vi "Reset Front Panel.vi"(7 "Active Display":u16, 8 "error in":errorcluster, 9 "Pane Origin":T1[](array[typedef]), 10 "Front Panel Bounds":T2, 11 "VI Ref":refnum<vi>) -> (0 "error out":errorcluster, 3 "VI Ref":refnum<vi>)   [LabVIEW 2014]
doc: "<B>Copyright</B>: (c) 2015 MHWirth. All rights reserved.\n\nThis subVI retreive the front panel size and organization. \nThis can be called in \"Panel Resize\" event of the VI when action is maximized."
uses:
  <vilib>/Utility/miscctls.llb/LVRectTypeDef.ctl
  <vilib>/Utility/miscctls.llb/LVPointTypeDef.ctl
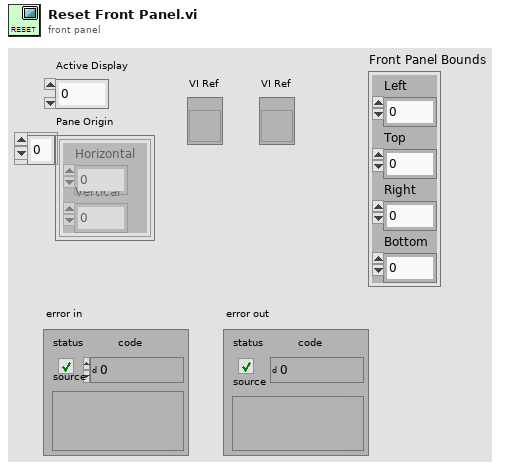
[diagram p1: front panel]
types:
  T1 = typedef "LVPointTypeDef.ctl" = cluster{"Horizontal":i16, "Vertical":i16}
  T2 = typedef "LVRectTypeDef.ctl" = cluster{"Left":i16, "Top":i16, "Right":i16, "Bottom":i16}
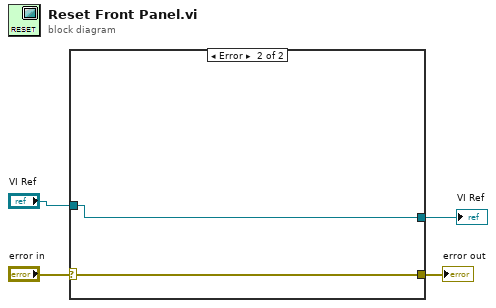
[diagram p0: block diagram]
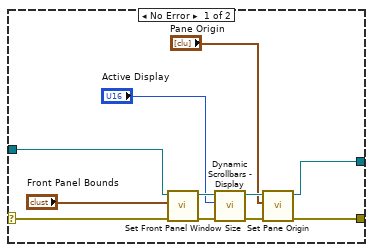
[diagram p2: hidden frame]
diagram:
  n1 = case shown="Error" "error in" {
    selector: "error in" -> [w11 w17]
    tunnel: [w10 w17] -> w3
    tunnel: "VI Ref" -> [w6 w16]
    tunnel: [w5 w16] -> w1
    frame No Error {
      n2 = call "Set Front Panel Window Size.vi"("error in"=w11, "Front Panel Window:Window Bounds"="Front Panel Bounds", "VI Ref"=w6) -> ("error out"=w15:errorcluster, "VI Ref"=w14:refnum<vi>)  [unwired: 7 in]
      n3 = call "Dynamic Scrollbars - Display.vi"("error in"=w15, "Active Display in"="Active Display", "VI Ref"=w14) -> ("error out"=w12:errorcluster, "VI Ref"=w13:refnum<vi>)  [unwired: 6 in, 1 out]
      n4 = call "Set Pane Origin.vi"("error in"=w12, "Pane Origin"="Pane Origin", "VI Ref"=w13) -> ("error out"=w10:errorcluster, "VI Ref"=w5:refnum<vi>)  [unwired: 7 in]
    }
    frame Error {
    }
  }
  "error out" <- w3
  "VI Ref" <- w1
